vi "libssh2_version - required version to high - returns empty string.vi"() -> ()   [LabVIEW 2013, in "libssh2_tests.lvlib"]
uses:
  libssh2_tests.lvlib
  libssh2/libssh2_init (Default).vi
  <vilib>/addons/_JKI Toolkits/Caraya/classes/Assert/Assert Equal Value_Variant.vi
  libssh2/libssh2.lvlib
  <vilib>/addons/_JKI Toolkits/Caraya/classes/Assert/Assert.lvclass
  <vilib>/addons/_JKI Toolkits/Caraya/classes/Test/Test.lvclass
panel:
  out "error out":errorcluster
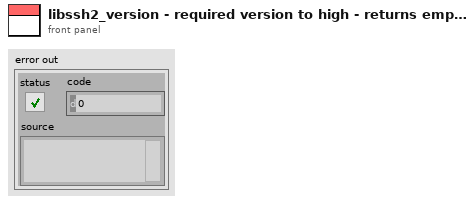
[diagram p1: front panel]
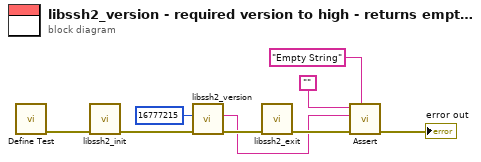
[diagram p0: block diagram]
diagram:
  n1 = call <vilib>:"Define Test.vi"() -> ("error out"=w5:errorcluster)  [unwired: 10 in, 1 out]
  n2 = call-poly "libssh2_init.vi"("error in (no error)"=w5) -> ("error out"=w9:errorcluster)  [unwired: 10 in]
  n3 = call "libssh2_version.vi"("error in (no error)"=w9, "required_version (0 = any)"=16777215) -> ("error out"=w7:errorcluster, "version"=w4:string)  [unwired: 8 in]
  n4 = call "libssh2_exit.vi"("error in (no error)"=w7) -> ("error out"=w8:errorcluster)  [unwired: 10 in]
  n5 = call-poly <vilib>:"Assert.vi"("Label"="Empty String", "error in (no error)"=w8, "Y"=w4, "X"="") -> ("error out"=→"error out":errorcluster)  [unwired: 6 in, 1 out]
